vi "locate enable tag.vi"(11 "data dictionary in":refnum<class "data dictionary.lvclass">) -> (1 "found?":bool, 2 "index":i32, 3 "data dictionary out":refnum<class "data dictionary.lvclass">)   [LabVIEW 2013, in "TDMS datalogger runtime.lvclass"]
uses:
  TDMS datalogger runtime.lvclass
  <vilib>/NI/Tag Bus/dictionary/data dictionary.lvclass
  <vilib>/NI/Tag Bus/dictionary/data dictionary.lvclass/data dictionary.ctl
  <vilib>/NI/Tag Bus/dictionary/lookup polymorphs/locate Boolean.vi
  <vilib>/NI/Tag Bus/dictionary/search/find data index.vi
  <vilib>/NI/Tag Bus/dictionary/search/search string list.vi
  <vilib>/NI/Tag Bus/dictionary/tag not found.vi
  configuration/TDMS datalogger configuration.lvclass
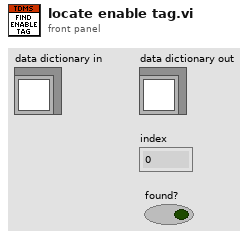
[diagram p1: front panel]
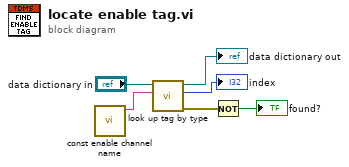
[diagram p0: block diagram]
diagram:
  n1 = call "const enable channel name.vi"() -> ("enable channel"=w3:string)  [unwired: 11 in]
  n2 = call-poly <vilib>:"look up tag by type.vi"("name"=w3, "data dictionary in"="data dictionary in") -> ("error out"=w6:errorcluster, "index"=→"index":i32, "data dictionary out"=→"data dictionary out":refnum<class "data dictionary.lvclass">)  [unwired: 7 in]
  n3 = Not(x=w6) -> (.not. x?=→"found?":bool)
